vi "InitDriverControl.vi"   [LabVIEW 2020]
doc: "This VI initializes user interface devices."
uses:
  <vilib>/Rock Robotics/WPI/Joystick/WPI_JoystickDeviceEnum.ctl
  refnums.vi
types:
  T1 = typedef "WPI_JoystickDeviceEnum.ctl" = enum16{"USB 0", "USB 1", "USB 2", "USB 3", "USB 4", "USB 5"}
  T2 = typedef "WPI_JoystickDevRef.ctl" = cluster{"Device":T1}
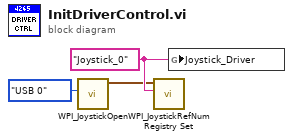
[diagram p0: block diagram]
diagram:
  w3 = "Joystick_0" ("Joystick_0")
  n1 = call <vilib>:"WPI_JoystickOpen.vi"("JoystickDevice"=WPI_JoystickDeviceEnum."USB 0") -> ("JoystickDevRef"=w2:T2)  [unwired: 10 in]
  n2 = call <vilib>:"WPI_JoystickRefNum Registry Set.vi"("refnum name"=w3, "JoystickDevRef"=w2) -> ()  [unwired: 8 in, 2 out]
  n3 = global write "refnums.vi" "Joystick_Driver"(w3) -> ()
